vi "Tree_Select first or last item.vi"(7 "Select Item":enum16{"First", "Last"}(ring), 8 "error in (no error)":errorcluster, 10 "Done Ref":refnum<vi>, 11 "Tree Ref":refnum<vi>) -> (0 "error out":errorcluster, 3 "Tree Ref Out":refnum<vi>)   [LabVIEW 2023]
doc: "If last and down, go to first; if first and up, go to last.\n\nTabbing to tree won't work if tree is empty, so if tree is empty on tab, go to Done."
panel:
  in  "Tree":string[](tree)
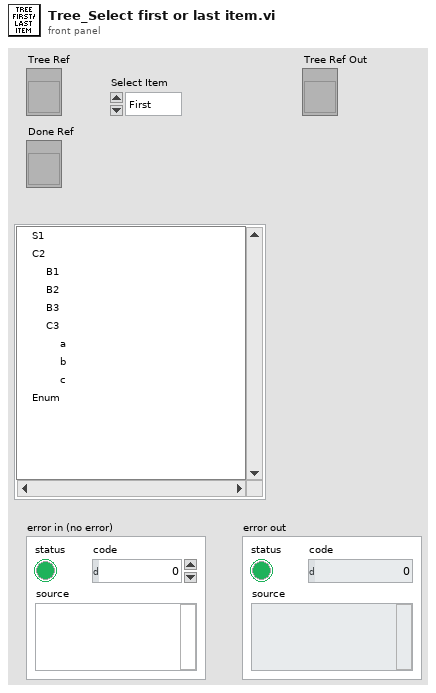
[diagram p1: front panel]
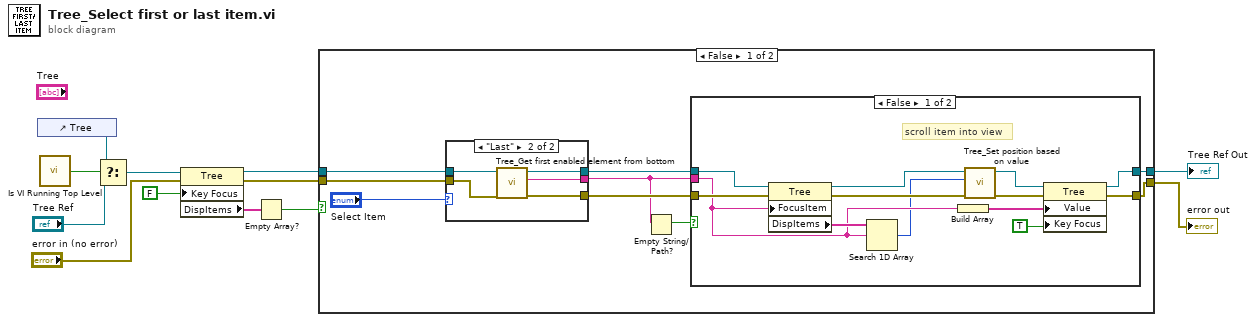
[diagram p0: block diagram]
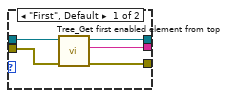
[diagram p3: hidden frame]
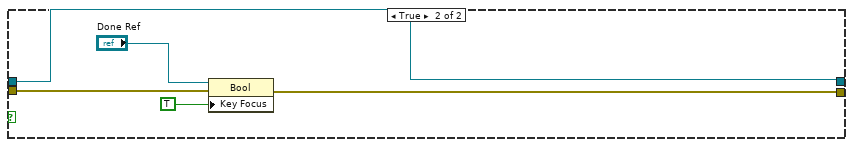
[diagram p4: hidden frame]
diagram:
  n1 = control-ref of="Tree"() -> (w11:refnum<vi>)
  n2 = call "Is VI Running Top Level.vi"() -> ("Top Level?"=w12:bool)  [unwired: 5 in]
  n3 = Select(t=w11, s=w12, f="Tree Ref") -> (s? t:f=w10:refnum<vi>)
  n4 = property class="Tree"(reference=w10, error in="error in (no error)", "Key Focus"=FALSE) -> (reference out=w6:refnum<vi>, error out=w4:errorcluster, "DispItems"=w2:string[])
  n5 = Empty Array?(array=w2) -> (empty?=w1:bool)
  n6 = case shown="False" w1 {
    tunnel: [w20 w47] -> w7
    tunnel: w6 -> [w19 w47]
    tunnel: w4 -> [w17 w51]
    tunnel: [w15 w48] -> w3
    frame False {
      n7 = case shown="\"Last\"" "Select Item" {
        tunnel: [w39 w44] -> w14
        tunnel: w19 -> [w41 w46]
        tunnel: [w40 w45] -> w18
        tunnel: w17 -> [w38 w43]
        tunnel: [w37 w42] -> w16
        frame "First", Default {
          n8 = call "Tree_Get first enabled element from top.vi"("error in (no error)"=w38, "Tree Control Ref"=w41) -> ("error out"=w37:errorcluster, "First Enabled Element"=w39:string, "Tree Control Ref Out"=w40:refnum<vi>)  [unwired: 7 in]
        }
        frame "Last" {
          n9 = call "Tree_Get first enabled element from bottom.vi"("error in (no error)"=w43, "TreeControl Ref"=w46) -> ("error out"=w42:errorcluster, "First Element Tag"=w44:string, "Tree Control Ref Out"=w45:refnum<vi>)  [unwired: 7 in]
        }
      }
      n10 = Empty String/Path?(string/path=w14) -> (empty?=w13:bool)
      n11 = case shown="False" w13 {
        tunnel: [w32 w36] -> w20
        tunnel: w18 -> [w31 w36]
        tunnel: w16 -> [w29 w35]
        tunnel: w14 -> [w25 _]
        tunnel: [w22 w35] -> w15
        frame False {
          # "scroll item into view"
          n12 = property class="Tree"(reference=w31, error in=w29, "FocusItem"=w25) -> (reference out=w30:refnum<vi>, error out=w28:errorcluster, "DispItems"=w26:string[])
          n13 = Search 1D Array(1D array=w26, element=w25) -> (index of element=w24:i32)  [unwired: 1 in]
          n14 = Build Array(w25) -> (w23:string[])
          n15 = call "Tree_Set position based on value.vi"("error in (no error)"=w28, "Selected Row"=w24, "Tree Ref"=w30) -> ("error out"=w27:errorcluster, "Tree Ref"=w33:refnum<vi>)  [unwired: 7 in]
          n16 = property class="Tree"(reference=w33, error in=w27, "Value"=w23, "Key Focus"=TRUE) -> (reference out=w32:refnum<vi>, error out=w22:errorcluster)
        }
        frame True {
        }
      }
    }
    frame True {
      n17 = property class="Bool"(reference="Done Ref", error in=w51, "Key Focus"=TRUE) -> (error out=w48:errorcluster)  [unwired: 1 out]
    }
  }
  "Tree Ref Out" <- w7
  "error out" <- w3
